vi "StageType.vi"(3 "Host address":string, 4 "Function":T1(ring), 5 "Stage Type (input)":T2) -> (0 "Host address (out)":string, 1 "VI Path":path, 2 "Stage Type (output)":T2 caption="Stage Setup (output)")   [LabVIEW 2009]
uses:
  StageType.ctt
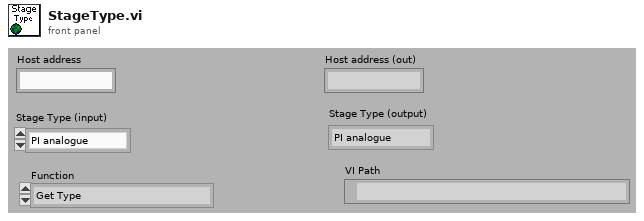
[diagram p1: front panel]
types:
  T1 = enum16{"Get Type", "Set Type", "GetStageInit", "GetWriteStageSetting", "GetInitializeStageOutput", "GetSetAxisPosition", "GetSetPos", "GetSetupStage", "HaltStageOutput", "InitializeStageOutputChannels"}
  T2 = typedef "StageType.ctt" = enum16{"PI analogue", "PI 712 TCP/IP", "Märzhäuser", "PI analogue step"}
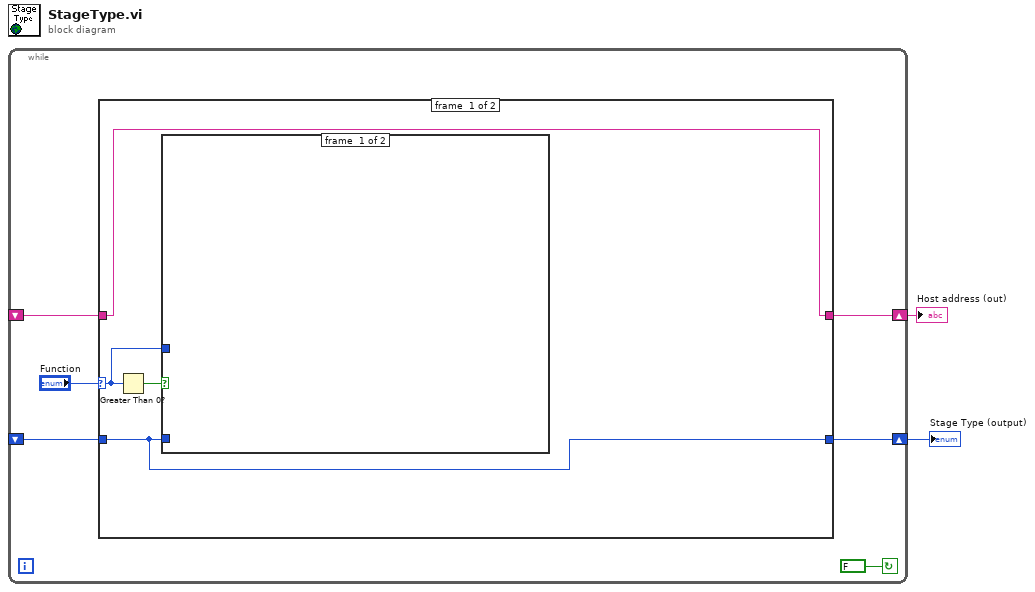
[diagram p0: block diagram]
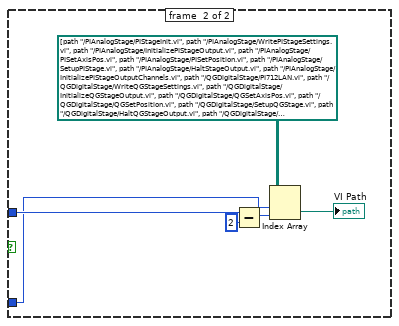
[diagram p2: hidden frame]
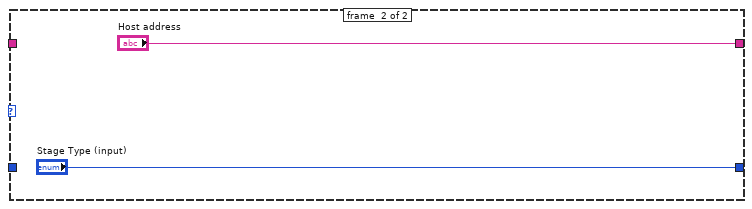
[diagram p3: hidden frame]
diagram:
  n1 = while {
    shift-right: [w5] -> w2
    shift-left: _ -> [w6]
    shift-right: [w4] -> w1
    shift-left: _ -> [w3]
    stop <- FALSE continue-if-true
    n2 = case shown="\"Get Type\", Default" "Function" {
      selector: "Function" -> [w10 _]
      tunnel: w6 -> [w11 _]
      tunnel: [w11 "Stage Type (input)"] -> w5
      tunnel: [w9 "Host address"] -> w4
      tunnel: w3 -> [w9 _]
      frame #0 {
        n3 = Greater Than 0?(x=w10) -> (x > 0?=w12:bool)
        n4 = case shown="True" w12 {
          tunnel: w11 -> [_ w14]
          tunnel: w10 -> [_ w17]
          frame #0 {
          }
          frame #1 {
            n5 = Subtract(x=w17, y=2) -> (x-y=w15:i32)
            n6 = Index Array(array=path[][] [[path "../PIAnalogStage/PIStageInit.vi", path "../PIAnalogStage/WritePIStageSettings.vi", path "../PIAnalogStage/InitializePIStageOutput.vi", path "../PIAnalogStage/PISetAxisPos.vi", path "../PIAnalogStage/PISetPosition.vi", path "../PIAnalogStage/SetupPIStage.vi", path "../PIAnalogStage/HaltStageOutput.vi", path "../PIAnalogStage/InitializePIStageOutputChannels.vi"], [path "../QGDigitalStage/PI712LAN.vi", path "../QGDigitalStage/WriteQGStageSettings.vi", path "../QGDigitalStage/InitializeQGStageOutput.vi", path "../QGDigitalStage/QGSetAxisPos.vi", path "../QGDigitalStage/QGSetPosition.vi", path "../QGDigitalStage/SetupQGStage.vi", path "../QGDigitalStage/HaltQGStageOutput.vi", path "../QGDigitalStage/InitializeQGStageOutputChannels.vi"], [path "../Märzhäuser/MWStageInit.vi", path "../Märzhäuser/WriteMWStageSettings.vi", path "../Märzhäuser/InitialzeMWStageOutput.vi", path "../Märzhäuser/MWSetAxisPos.vi", path "../Märzhäuser/MWSetPosition.vi", path "../Märzhäuser/SetupMWStage.vi", path "../Märzhäuser/HaltMWStageOutput.vi", path "../Märzhäuser/InitializeMWStageOutputChannels.vi"], [path "../PIAnalogStageTreppe/TPIStageInit.vi", path "../PIAnalogStageTreppe/TWritePIStageSettings.vi", path "../PIAnalogStageTreppe/TInitializePIStageOutput.vi", path "../PIAnalogStageTreppe/TPISetAxisPos.vi", path "../PIAnalogStageTreppe/TPISetPosition.vi", path "../PIAnalogStageTreppe/TSetupPIStage.vi", path "../PIAnalogStageTreppe/THaltStageOutput.vi", path "../PIAnalogStageTreppe/TInitializePIStageOutputChannels.vi"]] ("appended array"), index (row)=w14, index (col)=w15) -> (element=→"VI Path":path)
          }
        }
      }
      frame #1 {
      }
    }
  }
  "Stage Type (output)" <- w2
  "Host address (out)" <- w1
